vi "ATF-Pump NS Main.vi"(10 "Queues":T1, 11 "Pump DP":refnum<notifier>) -> ()   [LabVIEW 2022 SP3]
uses:
  Controls/SeCrTs-NS Data type.ctl
  UI Message handler/Message Queue/All Message Queues.ctl
  UI Message handler/Message Queue/Message Cluster.ctl
  UI Message handler/Message Queue/Message Queue.lvlib
panel:
  out "error out 2":errorcluster
  in  "error in 2":errorcluster
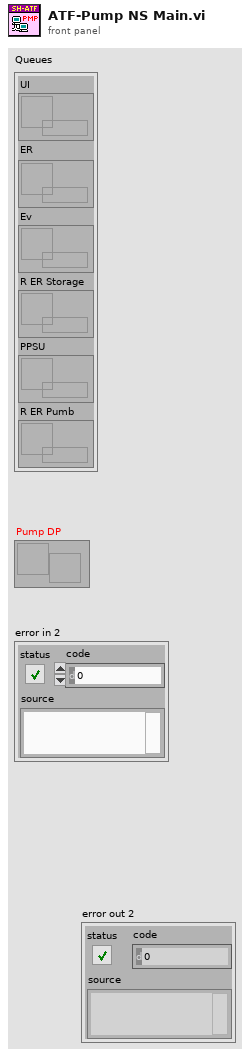
[diagram p1: front panel]
types:
  T1 = typedef "Message Queue.lvlib/All Message Queues.ctl" = cluster{"UI":refnum<queue>, "ER":refnum<queue>, "Ev":refnum<queue>, "R ER Storage":refnum<queue>, "PPSU":refnum<queue>, "R ER Pumb":refnum<queue>}
  T2 = cluster{"writer":refnum<k21>, "reader ":refnum<k21>, "Queues":T1}
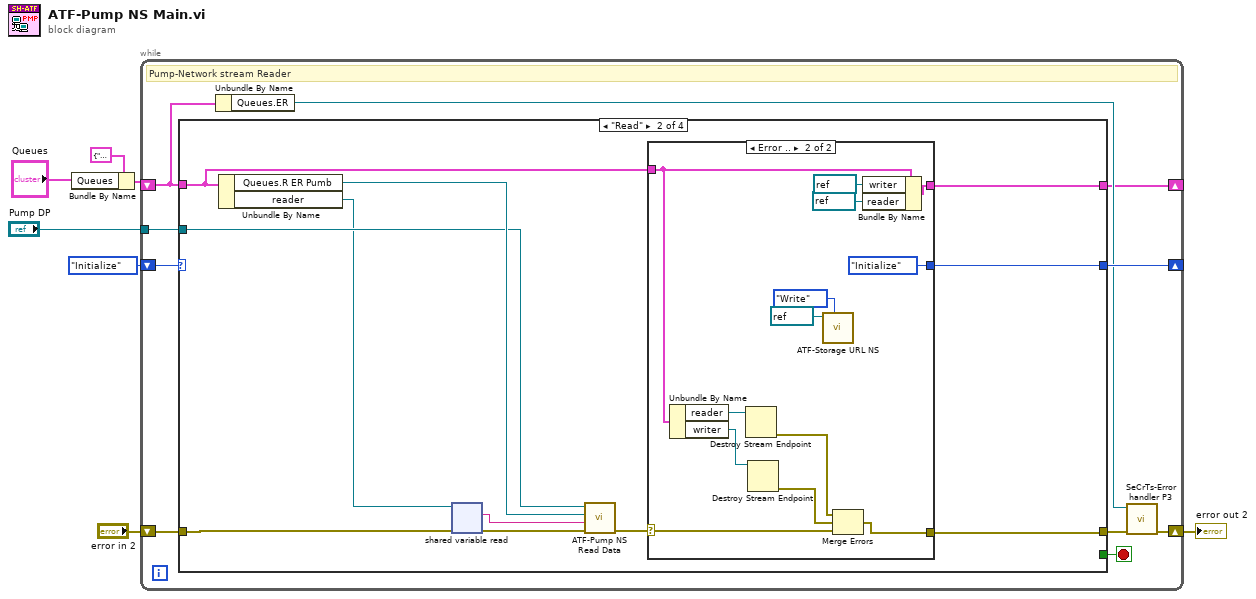
[diagram p0: block diagram]
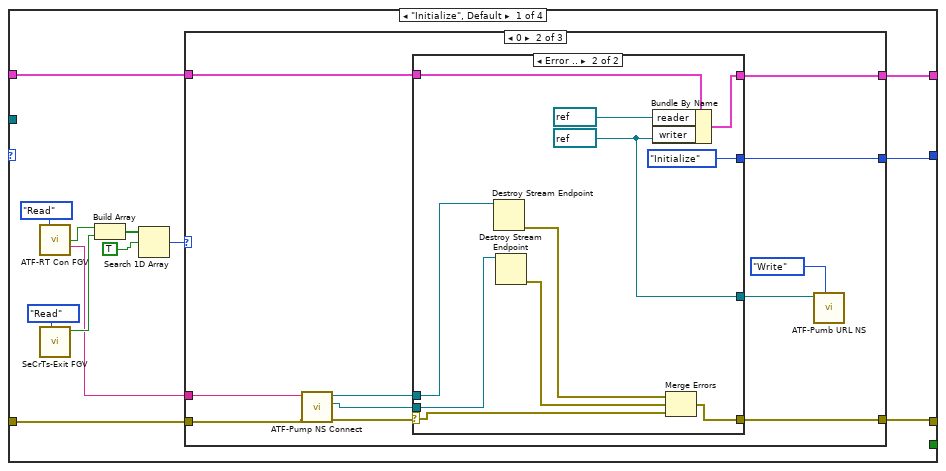
[diagram p2: hidden frame]
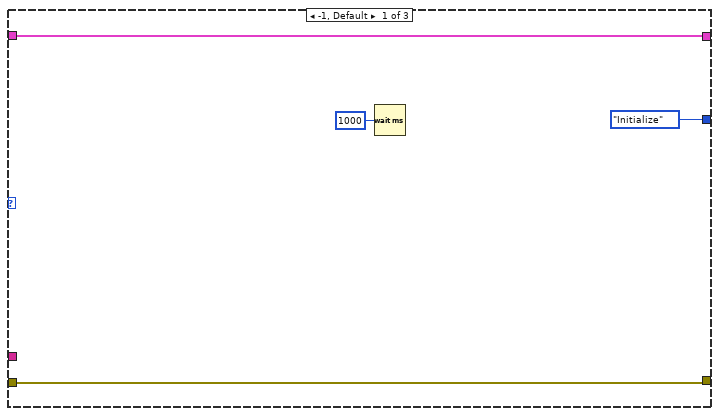
[diagram p3: hidden frame]
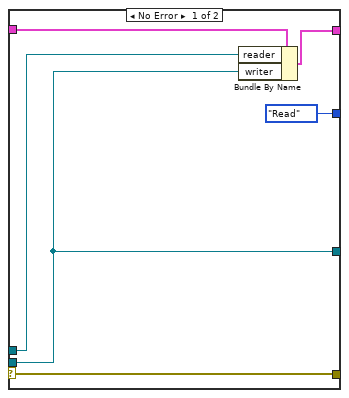
[diagram p4: hidden frame]
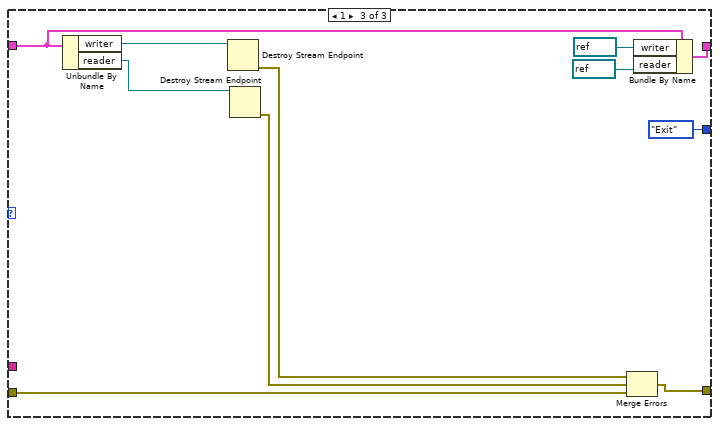
[diagram p5: hidden frame]
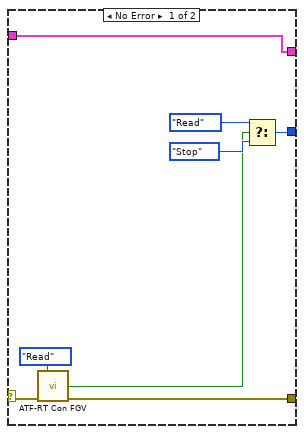
[diagram p6: hidden frame]
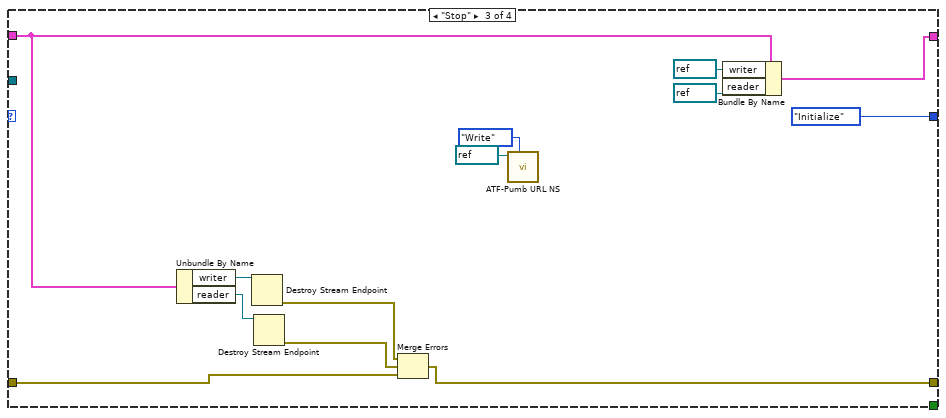
[diagram p7: hidden frame]
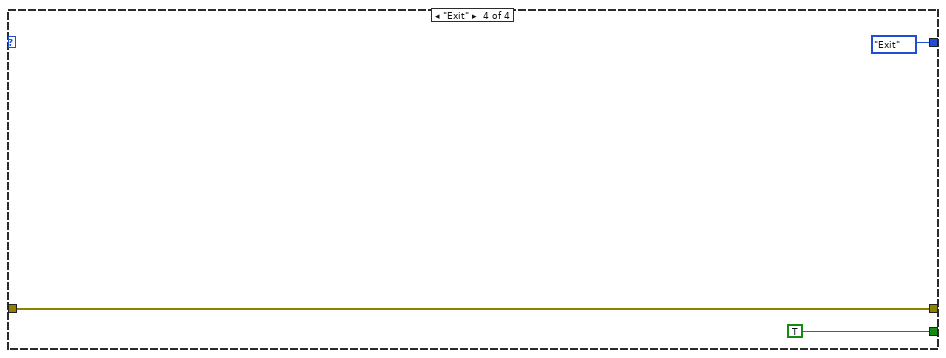
[diagram p8: hidden frame]
diagram:
  n1 = Bundle By Name(cluster=T2 {"writer"="", "reader "="", "Queues"={"UI"=refnum, "ER"=refnum, "Ev"=refnum, "R ER Storage"=refnum, "PPSU"=refnum, "R ER Pumb"=refnum}}, "Queues"="Queues") -> (w3:T2)
  n2 = while {
    shift-right: [w16] -> _
    shift-left: enum16{"Initialize", "Read", "Stop", "Exit"}."Initialize" -> [w17]
    tunnel: "Pump DP" -> [w15]
    shift-right: [w13] -> w4
    shift-left: "error in 2" -> [w14]
    shift-right: [w9] -> _
    shift-left: w3 -> [w11]
    stop <- w8 stop-if-true
    # "Pump-Network stream Reader"
    n3 = case shown="\"Read\"" w17 {
      tunnel: [w28 w76 enum16{"Initialize", "Read", "Stop", "Exit"}."Initialize" enum16{"Initialize", "Read", "Stop", "Exit"}."Exit"] -> w16
      tunnel: w15 -> [_ w83 _ _]
      tunnel: w14 -> [w23 w82 w113 w121]
      tunnel: [w22 w77 w114 w121] -> w12
      tunnel: w11 -> [w21 w74 w110 _]
      tunnel: [w20 w75 w117 _] -> w9
      tunnel: [_ _ _ TRUE] -> w8
      frame "Initialize", Default {
        n4 = call "ATF-RT Con FGV.vi"("Enum"=enum16{"Read", "Write"}."Read") -> ("Pumb rt con R"=w19:bool, "Pump IP R"=w18:string)  [unwired: 10 in, 3 out]
        n5 = call "SeCrTs-Exit FGV.vi"("Enum"=enum16{"Init", "Read", "Write"}."Read") -> ("Exit R"=w27:bool)  [unwired: 9 in, 1 out]
        n6 = Build Array(w19, w27) -> (w26:bool[])
        n7 = Search 1D Array(1D array=w26, element=TRUE) -> (index of element=w24:i32)  [unwired: 1 in]
        n8 = case shown="0" w24 {
          tunnel: [enum16{"Initialize", "Read", "Stop", "Exit"}."Initialize" w42 enum16{"Initialize", "Read", "Stop", "Exit"}."Exit"] -> w28
          tunnel: w23 -> [w31 w40 w68]
          tunnel: [w31 w43 w71] -> w22
          tunnel: w21 -> [w32 w45 w66]
          tunnel: [w32 w44 w67] -> w20
          tunnel: w18 -> [_ w41 _]
          frame -1, Default {
            n9 = Wait (ms)(milliseconds to wait=u32 1000) -> ()  [unwired: 1 out]
          }
          frame 0 {
            n10 = call "ATF-Pump NS Connect.vi"("error in (no error)"=w40, "Pump Ip Address"=w41) -> ("error out 2"=w39:errorcluster, "writer endpoint"=w38:refnum<k21>, "reader endpoint"=w37:refnum<k21>)  [unwired: 7 in]
            n11 = case shown="Error .." w39 {
              selector: w39 -> [w48 w57]
              tunnel: w45 -> [w51 w61]
              tunnel: [w50 w62] -> w44
              tunnel: w37 -> [w46 w60]
              tunnel: w38 -> [w47 w59]
              tunnel: [w48 w58] -> w43
              tunnel: [enum16{"Initialize", "Read", "Stop", "Exit"}."Read" enum16{"Initialize", "Read", "Stop", "Exit"}."Initialize"] -> w42
              tunnel: [w47 w52] -> w35
              frame No Error {
                n12 = Bundle By Name(cluster=w51, "reader"=w46, "writer"=w47) -> (w50:T2)
              }
              frame Error {
                w52 = refnum<k21> refnum ("writer")
                n13 = Destroy Stream Endpoint(11:w60) -> (0:w55:errorcluster)  [unwired: 1 in]
                n14 = Destroy Stream Endpoint(11:w59) -> (0:w56:errorcluster)  [unwired: 1 in]
                n15 = Bundle By Name(cluster=w61, "reader"=refnum<k21> refnum, "writer"=w52) -> (w62:T2)
                n16 = Merge Errors(w55, w56, w57) -> (w58:errorcluster)
              }
            }
            n17 = call "ATF-Pumb URL NS.vi"("Enum"=enum16{"Init", "Read", "Write"}."Write", "writer endpoint"=w35) -> ()  [unwired: 8 in, 2 out]
          }
          frame 1 {
            n18 = Unbundle By Name(w66) -> ("writer"=w73:refnum<k21>, "reader"=w72:refnum<k21>)
            n19 = Destroy Stream Endpoint(11:w73) -> (0:w70:errorcluster)  [unwired: 1 in]
            n20 = Destroy Stream Endpoint(11:w72) -> (0:w69:errorcluster)  [unwired: 1 in]
            n21 = Merge Errors(w70, w69, w68) -> (w71:errorcluster)
            n22 = Bundle By Name(cluster=w66, "writer"=refnum<k21> refnum, "reader"=refnum<k21> refnum) -> (w67:T2)
          }
        }
      }
      frame "Read" {
        n23 = Unbundle By Name(w74) -> ("Queues.R ER Pumb"=w84:refnum<queue>, "reader"=w81:refnum<k21>)
        n24 = shared-variable-read(w81, w82) -> (w80:errorcluster, w79:string)  [unwired: 1 in, 2 out]
        n25 = call "ATF-Pump NS Read Data.vi"("error in (no error)"=w80, "data"=w79, "Queues.R ER pump"=w84, "Notifier in"=w83) -> ("error out"=w78:errorcluster)  [unwired: 7 in]
        n26 = case shown="Error .." w78 {
          selector: w78 -> [w91 w93]
          tunnel: [w90 w96] -> w77
          tunnel: [w87 enum16{"Initialize", "Read", "Stop", "Exit"}."Initialize"] -> w76
          tunnel: [w86 w104] -> w75
          tunnel: w74 -> [w86 w99]
          frame No Error {
            n27 = call "ATF-RT Con FGV.vi"("Enum"=enum16{"Read", "Write"}."Read", "error in"=w91) -> ("Pumb rt con R"=w85:bool, "error out"=w90:errorcluster)  [unwired: 9 in, 3 out]
            n28 = Select(t=enum16{"Initialize", "Read", "Stop", "Exit"}."Read", s=w85, f=enum16{"Initialize", "Read", "Stop", "Exit"}."Stop") -> (s? t:f=w87:enum16{"Initialize", "Read", "Stop", "Exit"})
          }
          frame Error {
            n29 = Unbundle By Name(w99) -> ("reader"=w98:refnum<k21>, "writer"=w97:refnum<k21>)
            n30 = Destroy Stream Endpoint(11:w98) -> (0:w95:errorcluster)  [unwired: 1 in]
            n31 = Destroy Stream Endpoint(11:w97) -> (0:w94:errorcluster)  [unwired: 1 in]
            n32 = call "ATF-Storage URL NS.vi"("Enum"=enum16{"Init", "Read", "Write"}."Write", "writer endpoint"=refnum<k21> refnum) -> ()  [unwired: 8 in, 2 out]
            n33 = Merge Errors(w95, w94, w93) -> (w96:errorcluster)
            n34 = Bundle By Name(cluster=w99, "writer"=refnum<k21> refnum, "reader"=refnum<k21> refnum) -> (w104:T2)
          }
        }
      }
      frame "Stop" {
        n35 = Unbundle By Name(w110) -> ("writer"=w109:refnum<k21>, "reader"=w108:refnum<k21>)
        n36 = Destroy Stream Endpoint(11:w109) -> (0:w111:errorcluster)  [unwired: 1 in]
        n37 = Destroy Stream Endpoint(11:w108) -> (0:w112:errorcluster)  [unwired: 1 in]
        n38 = Merge Errors(w111, w112, w113) -> (w114:errorcluster)
        n39 = call "ATF-Pumb URL NS.vi"("Enum"=enum16{"Init", "Read", "Write"}."Write", "writer endpoint"=refnum<k21> refnum) -> ()  [unwired: 8 in, 2 out]
        n40 = Bundle By Name(cluster=w110, "writer"=refnum<k21> refnum, "reader"=refnum<k21> refnum) -> (w117:T2)
      }
      frame "Exit" {
      }
    }
    n41 = Unbundle By Name(w11) -> ("Queues.ER"=w10:refnum<queue>)
    n42 = call "SeCrTs-Error handler P3.vi"("error in"=w12, "Message Queue"=w10) -> ("error out"=w13:errorcluster)  [unwired: 8 in, 1 out]
  }
  "error out 2" <- w4
